vi "GyropFunc.vi"(6 "重置积分器":bool, 7 "error in (no error)":errorcluster, 10 "I2C Ref In":T1={"myRIO Reference"={"myRIO Model"=enum."Unknown", "myRIO Hardware Reference"={"Generic FPGA Reference"=refnum, "Allow multiple opens"=FALSE}}, "I2C Channels Enum"=enum."Not Connected", "I2C Configuration"={"I2C Transfer Rate"=enum."Fast mode (400 kbps)"}}) -> (0 "error":i32 caption="错误", 3 "转动的角度":dbl format="%0.2f")   [LabVIEW 2017]
uses:
  <vilib>/myRIO/Instrument Drivers/Onboard IO/I2C/typedefs/I2C Reference.ctl
  <vilib>/myRIO/Common/Instrument Driver Framework/Utilities/typedefs/myRIO Generic Hardware Reference.ctl
  <vilib>/myRIO/Common/Instrument Driver Framework/Utilities/typedefs/Hardware Version Enum.ctl
  <vilib>/myRIO/Common/Instrument Driver Framework/Utilities/typedefs/myRIO v1.0 Reference.ctl
  <vilib>/myRIO/Common/Instrument Driver Framework/Utilities/typedefs/Generic FPGA Reference.ctl
  <vilib>/myRIO/Common/Instrument Driver Framework/myRIO v1.0/I2C/typedefs/I2C Channels Enum.ctl
  <vilib>/myRIO/Instrument Drivers/Onboard IO/I2C/typedefs/I2C Configuration.ctl
  <vilib>/myRIO/Instrument Drivers/Onboard IO/I2C/typedefs/I2C Transfer Rate.ctl
  <vilib>/Utility/error.llb/Error Cluster From Error Code.vi
  <vilib>/myRIO/Common/Instrument Driver Framework/myRIO v1.0/I2C/vis/myRIO v1.0 Write I2C.vi
  <vilib>/myRIO/Common/Instrument Driver Framework/myRIO v1.0/I2C/vis/myRIO v1.0 Read I2C.vi
  <vilib>/myRIO/Instrument Drivers/Onboard IO/I2C/I2C.lvlib
  <vilib>/ptbypt/NI_PtbyPt.lvlib
panel:
  out "波形图表":i16(graph)
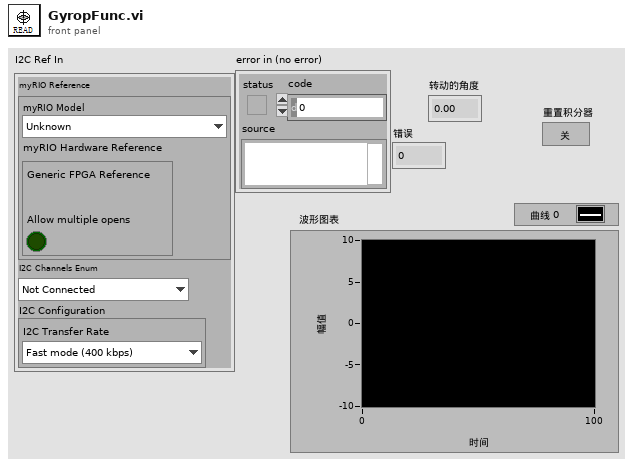
[diagram p1: front panel]
types:
  T1 = typedef "I2C.lvlib/I2C Reference.ctl" = cluster{"myRIO Reference":T2, "I2C Channels Enum":T6, "I2C Configuration":T7}
  T2 = typedef "myRIO Generic Hardware Reference.ctl" = cluster{"myRIO Model":T3, "myRIO Hardware Reference":T4}
  T3 = typedef "Hardware Version Enum.ctl" = enum16{"Unknown", "myRIO-1900", "myRIO-1950", "roboRIO", "NI ELVIS RIO CM"}
  T4 = typedef "myRIO v1.0 Reference.ctl" = cluster{"Generic FPGA Reference":T5, "Allow multiple opens":bool}
  T5 = typedef "Generic FPGA Reference.ctl" = refnum<k20>
  T6 = typedef "I2C Channels Enum.ctl" = enum16{"Not Connected", "A/I2C", "B/I2C", "I2C/I2C"}
  T7 = typedef "I2C.lvlib/I2C Configuration.ctl" = cluster{"I2C Transfer Rate":T8}
  T8 = typedef "I2C.lvlib/I2C Transfer Rate.ctl" = enum16{"Standard mode (100 kbps)", "Fast mode (400 kbps)"}
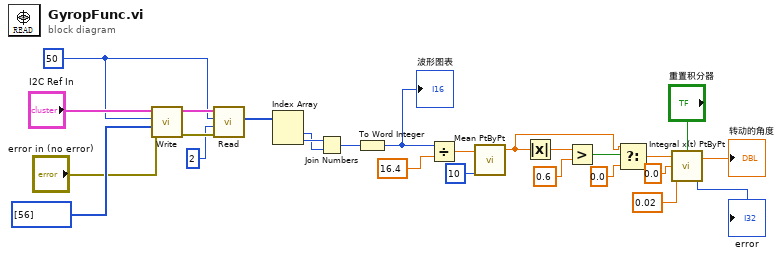
[diagram p0: block diagram]
diagram:
  w21 = u8 50 ("Slave Address (7-bit)")
  n1 = call <vilib>:"Write.vi"("error in (no error)"="error in (no error)", "Bytes to Write"=u8[] [56], "Slave Address (7-bit)"=w21, "I2C Ref In"="I2C Ref In") -> ("error out"=w23:errorcluster, "I2C Ref Out"=w22:T1)  [unwired: 6 in]
  n2 = call <vilib>:"Read.vi"("error in (no error)"=w23, "Byte Count"=u32 2, "Slave Address (7-bit)"=w21, "I2C Ref In"=w22) -> ("Bytes Read"=w19:u8[])  [unwired: 4 in, 2 out]
  n3 = Index Array(array=w19) -> (element #1=w17:u8, element #2=w18:u8)  [unwired: 2 in]
  n4 = Join Numbers(hi=w18, lo=w17) -> ((hi.lo)=w16:u16)
  n5 = To Word Integer(number=w16) -> (16bit integer=w14:i16)
  "波形图表" <- w14
  n6 = Divide(x=w14, y=16.4) -> (x/y=w13:dbl)
  n7 = call <vilib>:"Mean PtByPt.vi"("x"=w13, "sample length"=10) -> ("mean"=w8:dbl)  [unwired: 2 in, 1 out]
  n8 = Absolute Value(x=w8) -> (abs(x)=w11:dbl)
  n9 = Greater?(x=w11, y=0.6) -> (0:w9:bool)
  n10 = Select(t=w8, s=w9, f=0.0) -> (s? t:f=w6:dbl)
  n11 = call <vilib>:"Integral x(t) PtByPt.vi"("initialize"="重置积分器", "dt"=0.02, "initial condition"=0.0, "x"=w6) -> ("error"=→"error":i32, "integral x(t)"=→"转动的角度":dbl)
